vi "Serial Transmitter.vi"(10 "Porta:":refnum<visa-resource-name>, 11 "Robots":T1) -> (0 "error out":errorcluster)   [LabVIEW 2021]
uses:
  Convert AI Robot to Robot Command Folder/grSim/grSim Robot Command.ctl
  <vilib>/Instr/_visa.llb/VISA Configure Serial Port (Instr).vi
panel:
  out "return count":u32
  out "Array":u8[](array[numeric]) format="%02x"
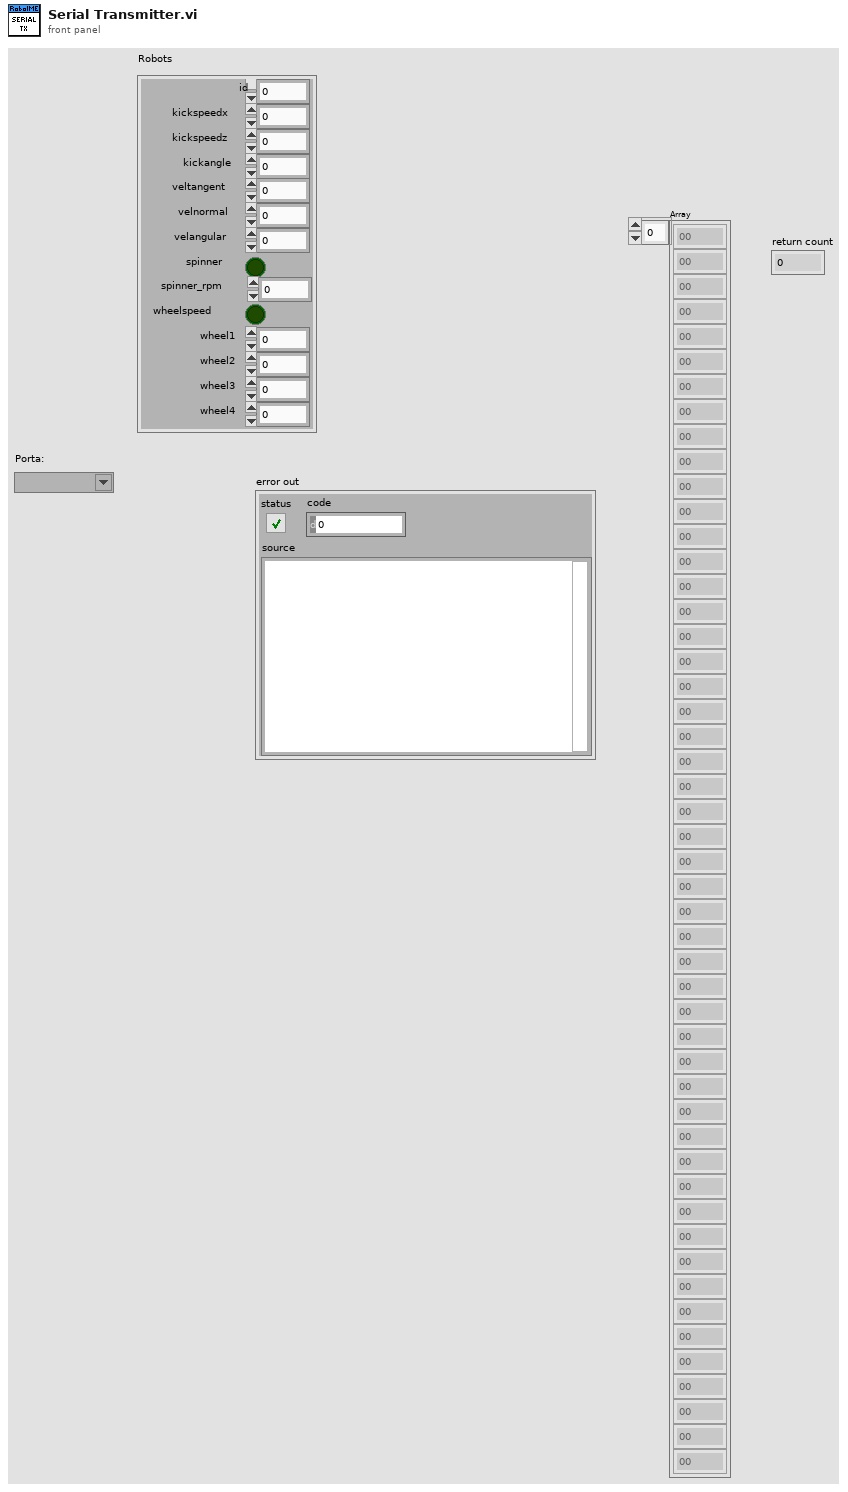
[diagram p1: front panel]
types:
  T1 = typedef "grSim Robot Command.ctl" = cluster{"id":u32, "kickspeedx":sgl, "kickspeedz":sgl, "veltangent":sgl, "velnormal":sgl, "velangular":sgl, "spinner":bool, "wheelspeed":bool, "wheel1":sgl, "wheel2":sgl, "wheel3":sgl, "wheel4":sgl, "kickangle":sgl, "spinner_rpm":sgl}
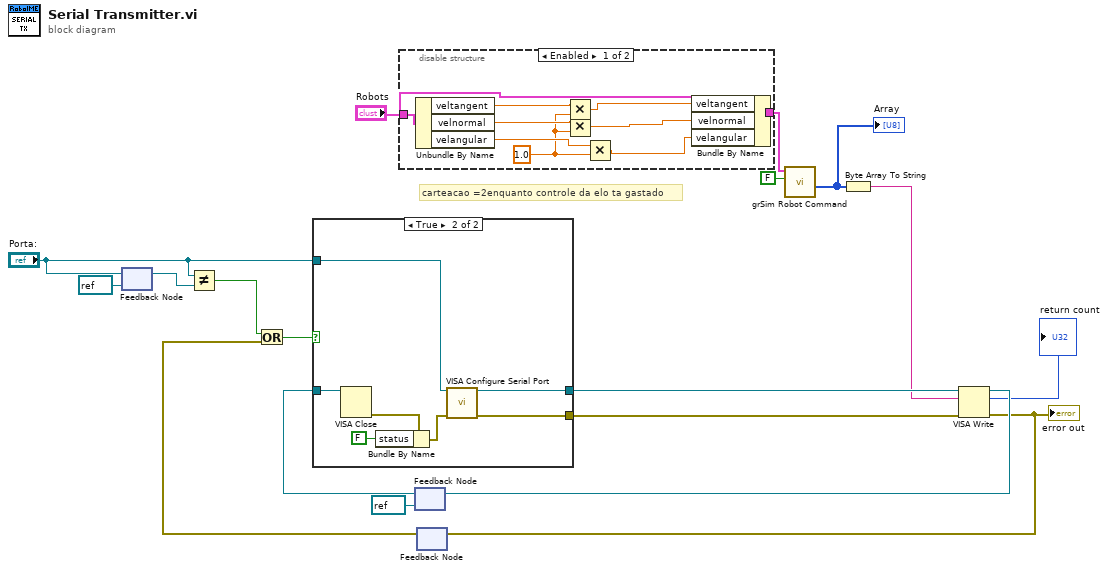
[diagram p0: block diagram]
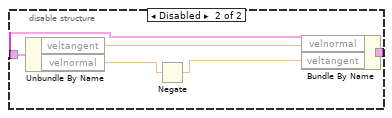
[diagram p2: hidden frame]
diagram:
  # "carteacao =2enquanto controle da elo ta gastado"
  n1 = feedback #1(refnum<visa-resource-name> refnum ("Porta?")) -> (w18:refnum<visa-resource-name>)
  n2 = feedback-in #1("Porta:") -> ()
  n3 = Not Equal?(x="Porta:", y=w18) -> (x != y?=w7:bool)
  n4 = disable-structure shown="Enabled" {
    disable-tunnel: "Robots" -> [w27 w32]
    disable-tunnel: [w26 w30] -> w3
    frame Enabled {
      w22 = 1.0
      n5 = Unbundle By Name(w27) -> ("veltangent"=w25:sgl, "velnormal"=w24:sgl, "velangular"=w23:sgl)
      n6 = Multiply(x=w25, y=w22) -> (x*y=w21:dbl)
      n7 = Multiply(x=w24, y=w22) -> (x*y=w20:dbl)
      n8 = Multiply(x=w23, y=w22) -> (x*y=w19:dbl)
      n9 = Bundle By Name(cluster=w27, "veltangent"=w21, "velnormal"=w20, "velangular"=w19) -> (w26:T1)
    }
    frame Disabled {
      n10 = Unbundle By Name(w32) -> ("veltangent"=w31:sgl, "velnormal"=w29:sgl)
      n11 = Negate(x=w29) -> (-x=w28:sgl)
      n12 = Bundle By Name(cluster=w32, "velnormal"=w31, "veltangent"=w28) -> (w30:T1)
    }
  }
  n13 = feedback #2(refnum<visa-resource-name> refnum ("VISA resource name out")) -> (w17:refnum<visa-resource-name>)
  n14 = feedback #3() -> (w6:errorcluster)  [unwired: 1 in]
  n15 = Or(x=w7, y=w6) -> (x .or. y?=w8:bool)
  n16 = case shown="True" w8 {
    tunnel: [_ w38] -> w13
    tunnel: [w33 w39] -> w14
    tunnel: "Porta:" -> [_ w34]
    tunnel: w17 -> [w33 w37]
    frame False {
    }
    frame True {
      n17 = VISA Close(VISA resource name=w37) -> (error out=w36:errorcluster)  [unwired: 1 in]
      n18 = Bundle By Name(cluster=w36, "status"=FALSE) -> (w35:errorcluster)
      n19 = call-poly "VISA Configure Serial Port"("VISA resource name"=w34, "error in (no error)"=w35) -> ("VISA resource name out"=w39:refnum<visa-resource-name>, "error out"=w38:errorcluster)  [unwired: 12 in]
    }
  }
  n20 = call "grSim Robot Command.vi"("FIRASim?"=FALSE, "Robots"=w3) -> ("Array"=w10:u8[])  [unwired: 9 in]
  "Array" <- w10
  n21 = Byte Array To String(unsigned byte array=w10) -> (string=w12:string)
  n22 = VISA Write(VISA resource name=w14, write buffer=w12, error in (no error)=w13) -> (VISA resource name out=w11:refnum<visa-resource-name>, return count=→"return count":u32, error out=w9:errorcluster)
  "error out" <- w9
  n23 = feedback-in #2(w11) -> ()
  n24 = feedback-in #3(w9) -> ()
